vi "q2.vi"() -> ()   [LabVIEW 2018]
uses:
  <vilib>/measure/NI_MABase.lvlib
panel:
  out "Meter":dbl(knob) scale=0.0..10.0
  in  "Knob":dbl(knob) scale=0.0..10.0
  in  "sampling info 2":cluster{"Fs":dbl, "#s":dbl}={"Fs"=1000.0, "#s"=1000.0} {"Fs" format="%.2p"}
  in  "phase":dbl format="%.2p"
  in  "frequency":dbl=10.0 format="%0.2p"
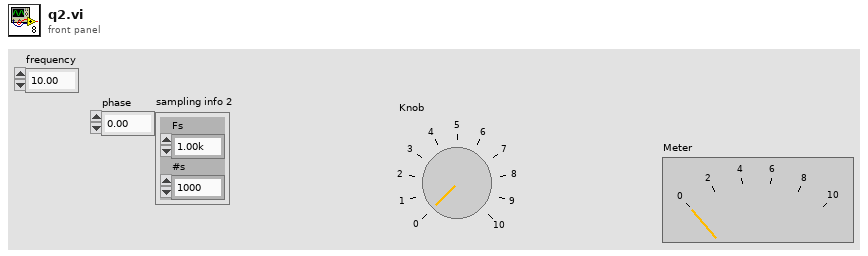
[diagram p1: front panel]
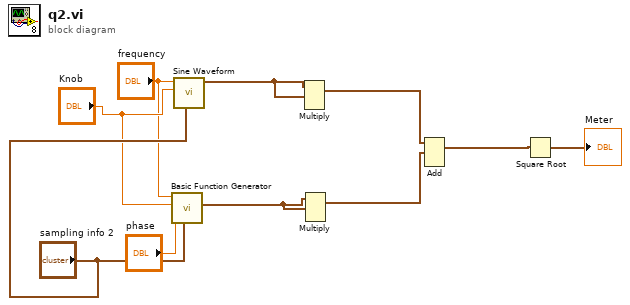
[diagram p0: block diagram]
diagram:
  n1 = call <vilib>:"Basic Function Generator.vi"("sampling info"="sampling info 2", "phase"="phase", "amplitude"="Knob", "frequency"="frequency") -> ("signal out"=w9:waveform(dbl))  [unwired: 5 in, 2 out]
  n2 = call <vilib>:"Sine Waveform.vi"("sampling info"="sampling info 2", "amplitude"="Knob", "frequency"="frequency") -> ("signal out"=w10:waveform(dbl))  [unwired: 7 in, 1 out]
  n3 = Multiply(1:w10, 2:w10) -> (0:w6:waveform(dbl))  [unwired: 1 in, 1 out]
  n4 = Multiply(1:w9, 2:w9) -> (0:w5:waveform(dbl))  [unwired: 1 in, 1 out]
  n5 = Add(1:w5, 2:w6) -> (0:w4:waveform(dbl))  [unwired: 1 in, 1 out]
  n6 = Square Root(x=w4) -> (sqrt(x)=→"Meter":waveform(dbl))
